vi "Hamamatsu_Init.vi"(0 "object in":refnum<class "Hamamatsu.lvclass">, 2 "Image Type":T1=7 items=["Grayscale (U8)", "Grayscale (I16)", "Grayscale (SGL)", "Complex (CSG)", "RGB (U32)", "HSL (U32)", "RGB (U64)", "Grayscale (U16)"], 5 "error in (no error)":errorcluster) -> (14 "object out":refnum<class "Hamamatsu.lvclass">, 19 "error out":errorcluster)   [LabVIEW 2021, in "Hamamatsu.lvclass"]
uses:
  Hamamatsu.lvclass
  Hamamatsu.lvclass/Hamamatsu.ctl
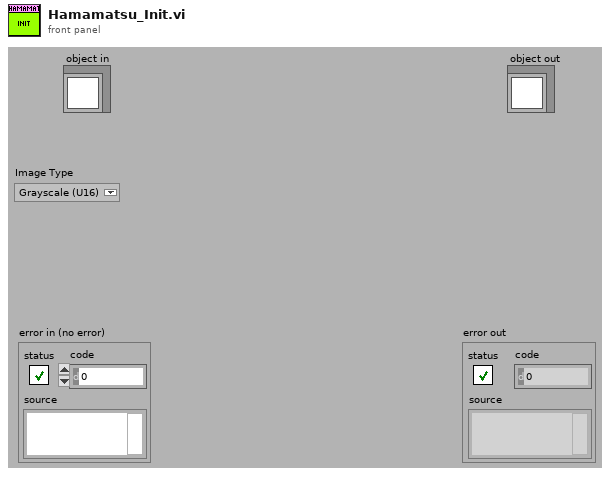
[diagram p1: front panel]
types:
  T1 = typedef "Image Type" = u32
  T2 = cluster{"Capture Library":string, "DCAM-API":string}
  T3 = typedef "IMAQ Image.ctl" = refnum<image>
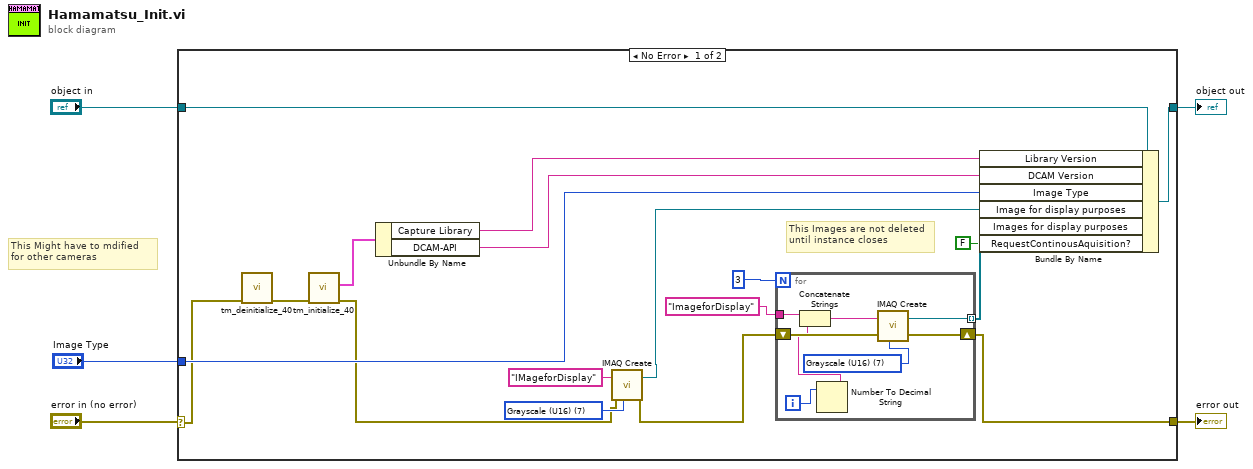
[diagram p0: block diagram]
diagram:
  # "This Might have to mdified \nfor other cameras"
  n1 = case shown="No Error" "error in (no error)" {
    selector: "error in (no error)" -> [w17 w32]
    tunnel: [w23 w33] -> w5
    tunnel: "object in" -> [w22 w33]
    tunnel: [w8 w32] -> w2
    tunnel: "Image Type" -> [w18 _]
    frame No Error {
      w13 = T1 7 items=["Grayscale (U8)", "Grayscale (I16)", "Grayscale (SGL)", "Complex (CSG)", "RGB (U32)", "HSL (U32)", "RGB (U64)", "Grayscale (U16)"] ("Image Type")
      # "This Images are not deleted\nuntil instance closes"
      n2 = call <userlib>:"tm_deinitialize_40.vi"("error in (no error)"=w17) -> ("error out"=w16:errorcluster)  [unwired: 10 in]
      n3 = call <userlib>:"tm_initialize_40.vi"("error in (no error)"=w16) -> ("error out"=w12:errorcluster, "Version Info"=w21:T2)  [unwired: 7 in, 2 out]
      n4 = Unbundle By Name(w21) -> ("Capture Library"=w20:string, "DCAM-API"=w19:string)
      n5 = call "IMAQ Create"("Image Name"="IMageforDisplay", "Image Type"=w13, "error in (no error)"=w12) -> ("New Image"=w14:T3, "error out"=w9:errorcluster)  [unwired: 2 in]
      n6 = for {
        N: 3 -> [_]
        tunnel: "ImageforDisplay" ("Image Name") -> [w31]
        shift-right: [w28] -> w8
        shift-left: w9 -> [w29]
        tunnel: [w26] -> w7 mode=indexing
        i -> [w24]
        w27 = T1 7 items=["Grayscale (U8)", "Grayscale (I16)", "Grayscale (SGL)", "Complex (CSG)", "RGB (U32)", "HSL (U32)", "RGB (U64)", "Grayscale (U16)"] ("Image Type")
        n7 = Number To Decimal String(number=w24) -> (decimal integer string=w25:string)  [unwired: 1 in]
        n8 = Concatenate Strings(w31, w25) -> (w30:string)
        n9 = call "IMAQ Create"("Image Name"=w30, "Image Type"=w27, "error in (no error)"=w29) -> ("New Image"=w26:T3, "error out"=w28:errorcluster)  [unwired: 2 in]
      }
      n10 = Bundle By Name(cluster=w22, "Library Version"=w20, "DCAM Version"=w19, "Image Type"=w18, "Image for display purposes"=w14, "Images for display purposes"=w7, "RequestContinousAquisition?"=FALSE) -> (w23:refnum<class "Hamamatsu.lvclass">)
    }
    frame Error {
    }
  }
  "object out" <- w5
  "error out" <- w2
